vi "writeToXML.vi"(8 "error in (no error)":errorcluster, 10 "Class Label":string, 11 "TCSCommand in":refnum<class "TCSCommand.lvclass">) -> (0 "error out":errorcluster, 2 "XML out":string, 3 "TCSCommand out":refnum<class "TCSCommand.lvclass">)   [LabVIEW 2014, in "TCSDataDefinitions.lvlib" / "TCSCommand.lvlib" / "TCSCommand.lvclass"]
uses:
  TCSCommand.lvclass
  TCSCommand.lvclass/TCSCommand.ctl
  <userlib>/Common/XML/XMLGenerator/XMLGenerator.lvclass
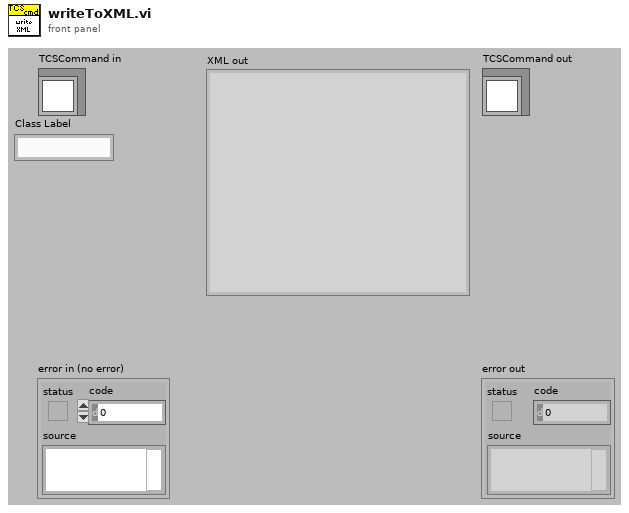
[diagram p1: front panel]
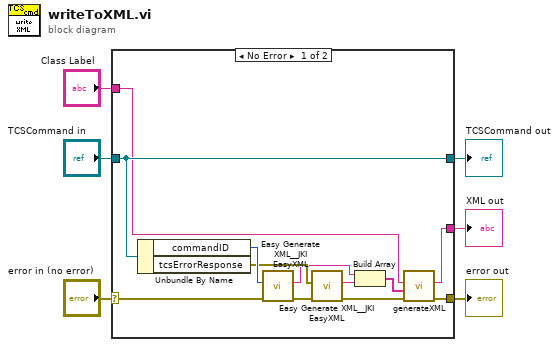
[diagram p0: block diagram]
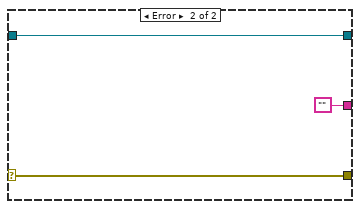
[diagram p2: hidden frame]
diagram:
  n1 = case shown="No Error" "error in (no error)" {
    selector: "error in (no error)" -> [w10 w21]
    tunnel: [w9 w21] -> w5
    tunnel: [w18 w20] -> w3
    tunnel: "TCSCommand in" -> [w18 w20]
    tunnel: "Class Label" -> [w8 _]
    tunnel: [w7 ""] -> w1
    frame No Error {
      n2 = Unbundle By Name(w18) -> ("commandID"=w17:u32, "tcsErrorResponse"=w16:errorcluster)
      n3 = call <vilib>:"Easy Generate XML__JKI EasyXML.vi"("error in (no error)"=w10, "LabVIEW Data"=w17) -> ("error out"=w15:errorcluster, "XML String"=w14:string)  [unwired: 8 in]
      n4 = call <vilib>:"Easy Generate XML__JKI EasyXML.vi"("error in (no error)"=w15, "LabVIEW Data"=w16) -> ("error out"=w11:errorcluster, "XML String"=w13:string)  [unwired: 8 in]
      n5 = Build Array(w14, w13) -> (w12:string[])
      n6 = call <userlib>:"generateXML.vi"("error in"=w11, "childrenXML"=w12, "elementName"=w8) -> ("error out"=w9:errorcluster, "XML out"=w7:string)  [unwired: 6 in, 1 out]
    }
    frame Error {
    }
  }
  "error out" <- w5
  "TCSCommand out" <- w3
  "XML out" <- w1
